vi "Build LEDs Section.vi"(6 "Cancelled?":bool, 8 "error in (no error)":errorcluster, 9 "Card Position in":T1 {"Slot #" max=15}, 10 "Name in":string, 11 "Node Ptr in":u64) -> (0 "error out":errorcluster)   [LabVIEW 2014, in "SLSC configuration System Explorer.lvlib"]
uses:
  SLSC configuration System Explorer.lvlib
  Type Defs/Card Position.ctl
  Shared/SPI Utility/Slot #.ctl
  <vilib>/NI Veristand/Custom Device API/Custom Device Channel.ctl
  <vilib>/NI Veristand/Custom Device API/Custom Device Channel Type.ctl
  Shared/Constants.vi
  <vilib>/NI Veristand/Custom Device API/Set Item Property (U16).vi
  <vilib>/NI Veristand/Custom Device API/Custom Device API.lvlib
  Shared/SLSC configuration Shared.lvlib
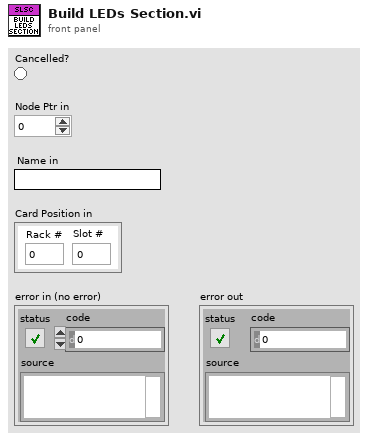
[diagram p1: front panel]
types:
  T1 = typedef "SLSC configuration Shared.lvlib/Card Position.ctl" = cluster{"Rack #":u8, "Slot #":T2}
  T2 = typedef "SLSC configuration Shared.lvlib/Slot #.ctl" = u8
  T3 = typedef "Custom Device API.lvlib/Custom Device Channel Type.ctl" = enum16{"Input", "Output"}
  T4 = typedef "Custom Device API.lvlib/Custom Device Channel.ctl" = cluster{"Type":T3, "Units":string, "Default Value":dbl, "Faultable":bool, "Scalable":bool}
  T5 = typedef "Custom Device API.lvlib/Custom Device Item Ref.ctl" = u64
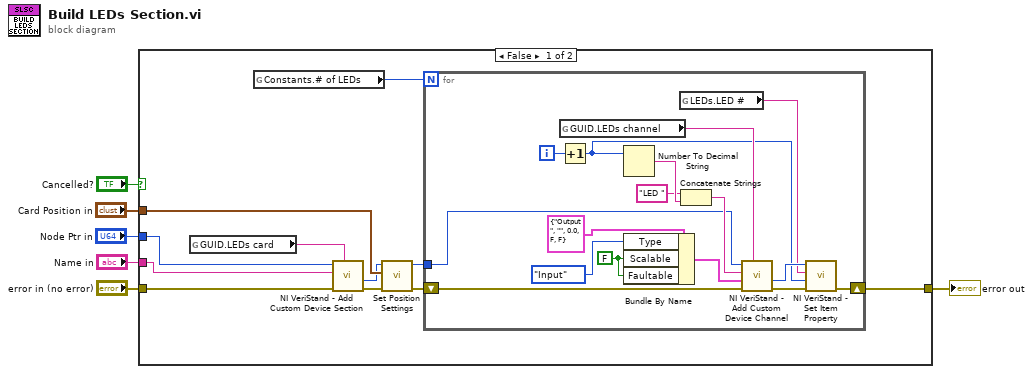
[diagram p0: block diagram]
diagram:
  n1 = case shown="False" "Cancelled?" {
    tunnel: "error in (no error)" -> [w17 w34]
    tunnel: "Node Ptr in" -> [w16 _]
    tunnel: "Card Position in" -> [w13 _]
    tunnel: [w7 w34] -> w5
    tunnel: "Name in" -> [w8 _]
    frame False {
      n2 = global read "Constants.vi" "GUID.LEDs card"() -> (w15:string)
      n3 = global read "Constants.vi" "Constants.# of LEDs"() -> (w11:u8)
      n4 = call <vilib>:"NI VeriStand - Add Custom Device Section.vi"("GUID (Default Section)"=w15, "error in (no error)"=w17, "Section Name"=w8, "Parent Ref in"=w16) -> ("error out"=w14:errorcluster, "Section Ptr"=w12:T5)  [unwired: 4 in, 2 out]
      n5 = call "Set Position Settings.vi"("error in (no error)"=w14, "Card Position"=w13, "Item Ref in"=w12) -> ("error out"=w10:errorcluster, "Item Ref out"=w9:T5)  [unwired: 7 in]
      n6 = for {
        N: w11 -> [_]
        shift-right: [w18] -> w7
        shift-left: w10 -> [w29]
        tunnel: w9 -> [w22]
        i -> [w28]
        w30 = FALSE ("Scalable")
        n7 = global read "Constants.vi" "GUID.LEDs channel"() -> (w24:string)
        n8 = Increment(x=w28) -> (x+1=w19:i32)
        n9 = Number To Decimal String(number=w19) -> (decimal integer string=w27:string)  [unwired: 1 in]
        n10 = Bundle By Name(cluster=T4 {"Type"=enum."Output", "Units"="", "Default Value"=0.0, "Faultable"=FALSE, "Scalable"=FALSE} ("Channel"), "Type"=Custom_Device_Channel_Type."Input", "Scalable"=w30, "Faultable"=w30) -> (w32:T4)
        n11 = global read "Constants.vi" "LEDs.LED #"() -> (w20:string)
        n12 = Concatenate Strings("LED " ("Channel Name"), w27) -> (w25:string)
        n13 = call <vilib>:"NI VeriStand - Add Custom Device Channel.vi"("GUID (Default Channel)"=w24, "error in (no error)"=w29, "Channel"=w32, "Channel Name"=w25, "Parent Ref in"=w22) -> ("error out"=w23:errorcluster, "Channel Ref"=w21:T5)  [unwired: 3 in, 2 out]
        n14 = call-poly <vilib>:"NI VeriStand - Set Item Property.vi"("error in (no error)"=w23, "Value"=w19, "Property Name"=w20, "Item Ref in"=w21) -> ("error out"=w18:errorcluster)  [unwired: 5 in, 2 out]
      }
    }
    frame True {
    }
  }
  "error out" <- w5
